vi "BME_DG_SetV2TriggerParameters.vi"(8 "error in (no error)":errorcluster, 10 "V2 Trigger Settings":T1={"Trigger on MS Bus"=24, "Force Trigger (µs)"=0.0, "Gate Type"=TRUE, "Synchronize Gate"=FALSE} {"Trigger on MS Bus" format="%04x" items=["Local Primary0x1"=1, "Local Secondary0x2"=2, "Local Force 0x4"=4, "Resynchronize 0x8"=8, "StepBackOnBus 0x10"=16, "StartOnBus 0x20"=32, "InhibitOnBus 0x40"=64, "LoadDataOnBus 0x80"=128]; "Force Trigger (µs)" min=0.0 format="%.6f"}, 11 "DG Number":i32) -> (0 "error out":errorcluster)   [LabVIEW 2009, in "POLARIS BME DG.lvlib"]
doc: "long Set_V2_TriggerParameters(BOOL IgnoreGate, BOOL SynchronizeGate, double ForceTrigger, \n unsigned long MS_Bus, long DG_Number);"
uses:
  POLARIS BME DG.lvlib
  BME_DG_V2TriggerSettings.ctl
  MSBusSignals.ctl
  BME DLL/DelayGenerator.dll
panel:
  # "NOTICE -- YOU MUST LEAVE THIS NOTICE IN PLACE.  PER THE TERMS OF THE LICENSE BELOW, YOU MAY SUBLICENSE THIS SOFTWARE \nIN ANY WAY THAT DOES NOT CONFLICT WITH THIS LICENSE.\n\n### BSD License (http://www.opensource.org/licenses/bsd-license.php) Begin ###\n \nCopyright (c) 2011, Applied Energetics, http://www.appliedenergetics.com,\n                               Richard Schwerdtfeger, <rschwerdtfeger@appliedenergetics.com>\n\nAll rights reserved.\n\nRedistribution and use in source and binary forms, with or without modification, are permitted provided that the \nfollowing conditions are met:\n\n    * Redistributions of source code must retain the above copyright notice, this list of conditions and the following disclaimer.\n    * Redistributions in binary form must reproduce the above copyright notice, this list of conditions and the following disclaimer \n       in the documentation and/or other materials provided with the distribution.\n    * Neither the name of Richard Schwerdtfeger, Applied Energetics, Inc., nor the names of its contributors may be used to \n       endorse or promote products derived from this software without specific prior written permission.\n\nTHIS SOFTWARE IS PROVIDED BY THE COPYRIGHT HOLDERS AND CONTRIBUTORS \"AS IS\" AND ANY EXPRESS OR IMPLIED WARRANTIES, \nINCLUDING, BUT NOT LIMITED TO, THE IMPLIED WARRANTIES OF MERCHANTABILITY AND FITNESS FOR A PARTICULAR PURPOSE ARE \nDISCLAIMED. IN NO EVENT SHALL THE COPYRIGHT OWNER OR CONTRIBUTORS BE LIABLE FOR ANY DIRECT, INDIRECT, INCIDENTAL,\n SPECIAL, EXEMPLARY, OR CONSEQUENTIAL DAMAGES (INCLUDING, BUT NOT LIMITED TO, PROCUREMENT OF SUBSTITUTE GOODS OR \nSERVICES; LOSS OF USE, DATA, OR PROFITS; OR BUSINESS INTERRUPTION) HOWEVER CAUSED AND ON ANY THEORY OF LIABILITY, \nWHETHER IN CONTRACT, STRICT LIABILITY, OR TORT (INCLUDING NEGLIGENCE OR OTHERWISE) ARISING IN ANY WAY OUT OF THE USE \nOF THIS SOFTWARE, EVEN IF ADVISED OF THE POSSIBILITY OF SUCH DAMAGE.\n\n### BSD License End ###"
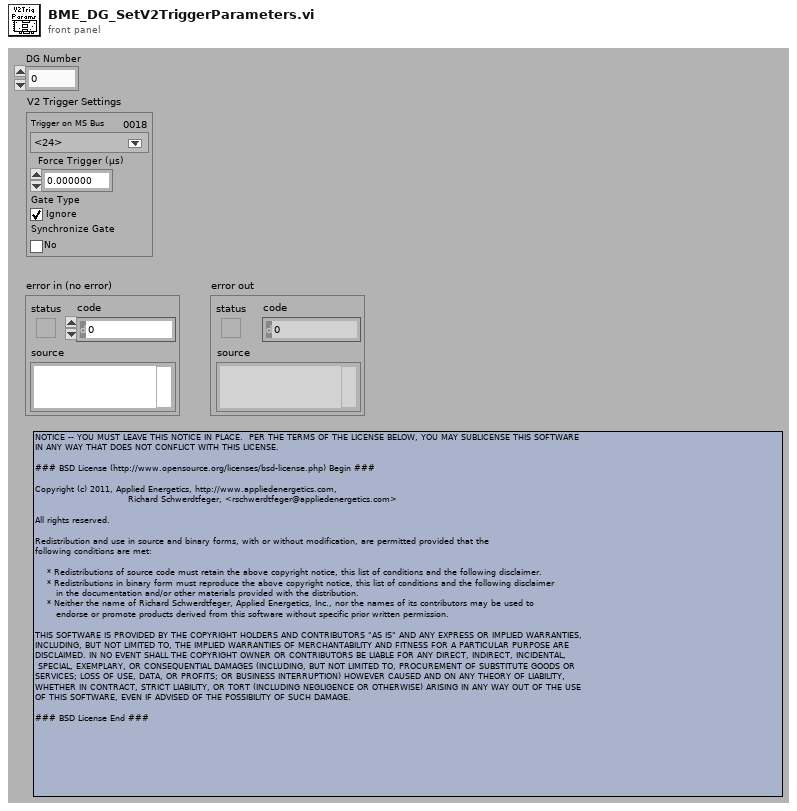
[diagram p1: front panel]
types:
  T1 = typedef "POLARIS BME DG.lvlib/BME_DG_V2TriggerSettings.ctl" = cluster{"Trigger on MS Bus":T2, "Force Trigger (µs)":dbl, "Gate Type":bool, "Synchronize Gate":bool}
  T2 = typedef "POLARIS BME DG.lvlib/MSBusSignals.ctl" = u32
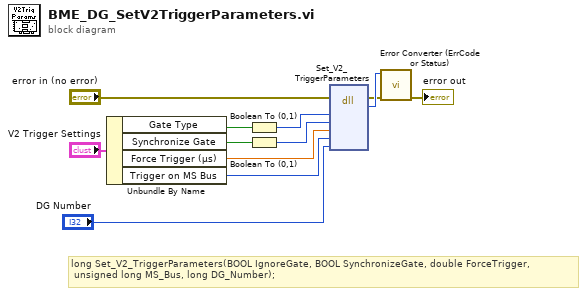
[diagram p0: block diagram]
diagram:
  # "long Set_V2_TriggerParameters(BOOL IgnoreGate, BOOL SynchronizeGate, double ForceTrigger, \n unsigned long MS_Bus, long DG_Number);"
  n1 = Unbundle By Name("V2 Trigger Settings") -> ("Gate Type"=w4:bool, "Synchronize Gate"=w3:bool, "Force Trigger (µs)"=w2:dbl, "Trigger on MS Bus"=w1:T2)
  n2 = Boolean To (0,1)(Boolean=w4) -> (0, 1=w7:i16)
  n3 = Boolean To (0,1)(Boolean=w3) -> (0, 1=w6:i16)
  n4 = dll-call lib="D:/CS Framework/LVSCC/LV2009/GPL/Projects/cs-framework/CSClass/CSPOLARIS/POLARIS BME DG/BME DLL/DelayGenerator.*" fn="Set_V2_TriggerParameters"(error in="error in (no error)", "IgnoreGate"=w7, "SynchronizeGate"=w6, "ForceTrigger"=w2, "MS_Bus"=w1, "DG_Number"="DG Number") -> (error out=w9:errorcluster, w12:i32)  [unwired: 5 in, 3 out]
  n5 = call "Error Converter (ErrCode or Status).vi"("error in (no error)"=w9, "error code"=w12) -> ("error out"=→"error out":errorcluster)  [unwired: 9 out]
